vi "test.vi"() -> ()   [LabVIEW 2016]
uses:
  DataTypes/logevent_DetailedState.ctl
  SALLV_EXA.lvlib
panel:
  out "logevent_DetailedState_Ctl out":T1
  out "x+1":i32
  in  "Boolean":bool
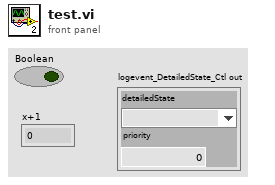
[diagram p1: front panel]
types:
  T1 = typedef "SALLV_EXA.lvlib/logevent_DetailedState.ctl" = cluster{"detailedState":enum16{"", " DisabledState", "EnabledState", "FaultState", "OfflineState", "StandbyState"}, "priority":i32}
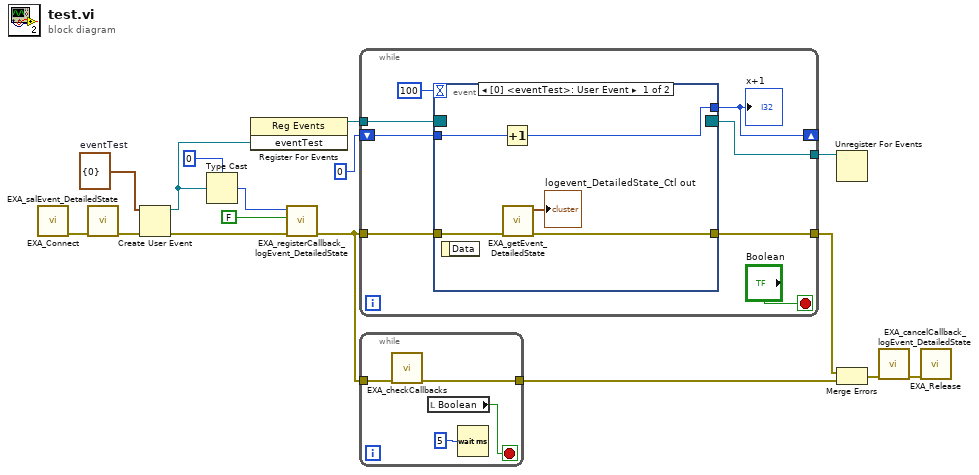
[diagram p0: block diagram]
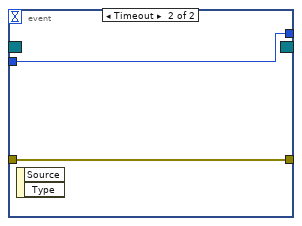
[diagram p2: hidden frame]
diagram:
  w8 = cluster{"Data":i32} {"Data"=0}  # eventTest
  n1 = call "EXA_Connect.vi"() -> ("error out"=w11:errorcluster)  [unwired: 10 in, 1 out]
  n2 = call "EXA_salEvent_DetailedState.vi"("error in (no error)"=w11) -> ("error out"=w2:errorcluster)  [unwired: 9 in, 1 out]
  n3 = Create User Event(user event datatype=w8, error in=w2) -> (user event=w4:refnum<user-event>, error out=w1:errorcluster)
  n4 = Type Cast(type=0 ("handle"), x=w4) -> (*(type *) &x=w6:i32)
  n5 = register-events(w4) -> (reference out=w10:refnum<event-registration>)  [unwired: 2 in, 1 out]
  n6 = call "EXA_registerCallback_logEvent_DetailedState.vi"("error in (no error)"=w1, "skipOld"=FALSE, "handle"=w6) -> ("error out"=w3:errorcluster)  [unwired: 7 in, 1 out]
  n7 = while {
    tunnel: [w23] -> w13
    shift-right: [w17] -> _
    shift-left: 0 -> [w18]
    tunnel: w10 -> [w22]
    tunnel: [w21] -> w9
    tunnel: w3 -> [w20]
    stop <- "Boolean" stop-if-true
    n8 = event shown="[0] <eventTest>: User Event" {
      selector: w22 -> [_ _]
      dyn-events: [_ _] -> w21
      timeout: 100 -> [_ _]
      tunnel: [w29 w31] -> w23
      tunnel: w20 -> [w27 w31]
      tunnel: w18 -> [w26 w30]
      tunnel: [w25 w30] -> w17
      event User Event {
        n9 = event-data() -> ()  [unwired: 1 in, 1 out]
        n10 = Increment(x=w26) -> (x+1=w25:i32)
        n11 = call "EXA_getEvent_DetailedState.vi"("error in (no error)"=w27) -> ("error out"=w29:errorcluster, "logevent_DetailedState_Ctl out"=→"logevent_DetailedState_Ctl out":T1)  [unwired: 8 in, 1 out]
      }
      event Timeout {
        n12 = event-data() -> ()  [unwired: 1 in, 2 out]
      }
    }
    "x+1" <- w17
  }
  n13 = while {
    tunnel: [w33] -> w14
    tunnel: w3 -> [w32]
    stop <- w34 stop-if-true
    n14 = call "EXA_checkCallbacks.vi"("error in (no error)"=w32) -> ("error out"=w33:errorcluster)  [unwired: 10 in]
    n15 = local read "Boolean"() -> (w34:bool)
    n16 = Wait (ms)(milliseconds to wait=u32 5) -> ()  [unwired: 1 out]
  }
  n17 = Unregister For Events(event registration refnum=w9) -> ()  [unwired: 1 in, 1 out]
  n18 = Merge Errors(w13, w14) -> (w15:errorcluster)
  n19 = call "EXA_cancelCallback_logEvent_DetailedState.vi"("error in (no error)"=w15) -> ("error out"=w16:errorcluster)  [unwired: 9 in, 1 out]
  n20 = call "EXA_Release.vi"("error in (no error)"=w16) -> ()  [unwired: 9 in, 2 out]
